vi "fit slope data to exponential decay.vi"(10 "length":i32=1000, 11 "remaining elements":T1[](array[typedef])) -> (2 "graphs":cluster{dbl[], dbl[]}[](array[cluster]), 3 "lifetime":dbl)   [LabVIEW 2017]
uses:
  typedefs/reading1.ctl
  <vilib>/Analysis/NI_AALPro.lvlib
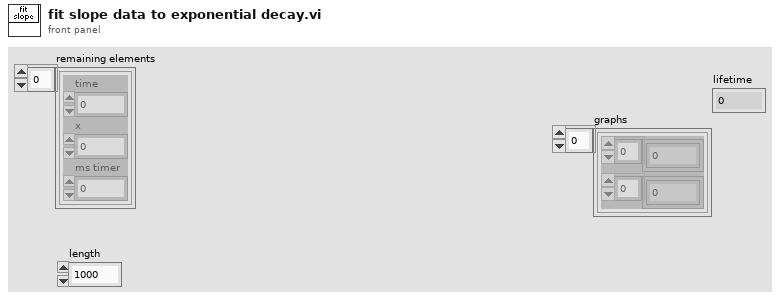
[diagram p1: front panel]
types:
  T1 = typedef "reading1.ctl" = cluster{"time":dbl, "x":dbl, "ms timer":u32}
  T2 = cluster{"amp min":dbl, "amp max":dbl, "damping min":dbl, "damping max":dbl, "offset min":dbl, "offset max":dbl}
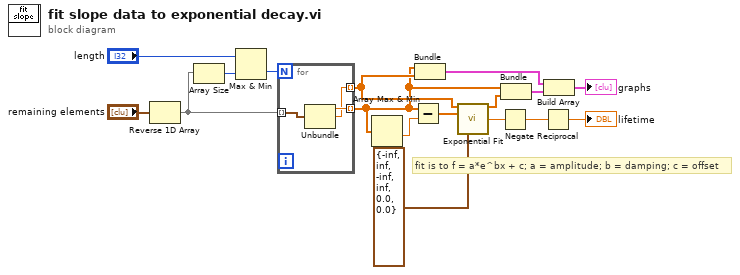
[diagram p0: block diagram]
diagram:
  # "fit is to f = a*e^bx + c; a = amplitude; b = damping; c = offset"
  n1 = Reverse 1D Array(array="remaining elements") -> (reversed array=w16:T1[])
  n2 = Array Size(array=w16) -> (size(s)=w15:i32)
  n3 = Max & Min(x="length", y=w15) -> (min(x,y)=w13:i32)  [unwired: 1 out]
  n4 = for {
    N: w13 -> [_]
    tunnel: w16 -> [w20] mode=indexing
    tunnel: [w19] -> w9 mode=indexing
    tunnel: [w18] -> w12 mode=indexing
    n5 = Unbundle(w20) -> ("time"=w19:dbl, "x"=w18:dbl)  [unwired: 1 out]
  }
  n6 = Array Max & Min(array=w9) -> (min value=w2:dbl)  [unwired: 3 out]
  n7 = Subtract(x=w9, y=w2) -> (x-y=w8:dbl[])
  n8 = Bundle(w9, w12) -> (w11:cluster{dbl[], dbl[]})  [unwired: 1 in]
  n9 = call <vilib>:"Exponential Fit.vi"("Y"=w12, "X"=w8, "parameter bounds"=T2 {"amp min"=-inf, "amp max"=inf, "damping min"=-inf, "damping max"=inf, "offset min"=0.0, "offset max"=0.0}) -> ("Best Exponential Fit"=w7:dbl[], "damping"=w6:dbl)  [unwired: 7 in, 4 out]
  n10 = Negate(x=w6) -> (-x=w5:dbl)
  n11 = Bundle(w9, "Best Exponential Fit"=w7) -> (w3:cluster{dbl[], "Best Exponential Fit":dbl[]})  [unwired: 1 in]
  n12 = Reciprocal(x=w5) -> (1/x=→"lifetime":dbl)
  n13 = Build Array(w11, w3) -> (→"graphs":cluster{dbl[], "Best Exponential Fit":dbl[]}[])
